vi "PantherLAB_Log - Add New DQMH Module.vi"(4 "New Module Name":string, 6 "New Module Folder":path, 9 "External Module Info":T1, 10 "New Module Type":T3, 11 "Project":refnum<vi>) -> (0 "error out":errorcluster)   [LabVIEW 2016]
doc: "_____\nCreated using DQMH Framework: Event Scripter 7.1.0.1450."
uses:
  <vilib>/Delacor/Delacor QMH/Libraries/_Scripting Support/Module Type (Including External)--enum.ctl
  <vilib>/Delacor/Delacor QMH/Libraries/_Scripting Support/External Module Info--cluster.ctl
  <vilib>/Delacor/Delacor QMH/Libraries/_Scripting Support/Module Type--enum.ctl
  PantherLAB Scripting Hooks/PantherLAB_Log.lvlib
  <vilib>/Delacor/Delacor QMH/Libraries/_Scripting Support/dqmh_lib_DQMH Scripting Support.lvlib
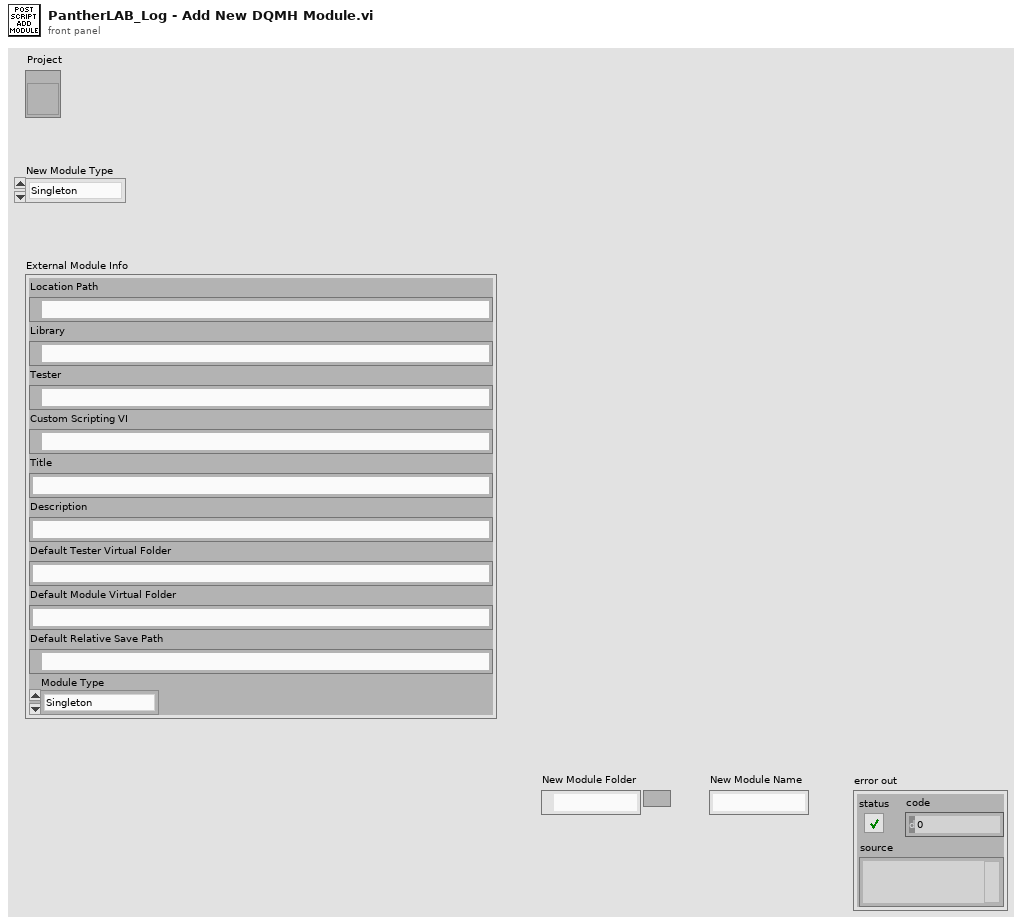
[diagram p1: front panel]
types:
  T1 = typedef "dqmh_lib_DQMH Scripting Support.lvlib/External Module Info--cluster.ctl" = cluster{"Location Path":path, "Library":path, "Tester":path, "Custom Scripting VI":path, "Title":string, "Description":string, "Default Tester Virtual Folder":string, "Default Module Virtual Folder":string, "Default Relative Save Path":path, "Module Type":T2}
  T2 = typedef "dqmh_lib_DQMH Scripting Support.lvlib/Module Type--enum.ctl" = enum16{"Singleton", "Cloneable"}
  T3 = typedef "dqmh_lib_DQMH Scripting Support.lvlib/Module Type (Including External)--enum.ctl" = enum16{"Singleton", "Cloneable", "External"}
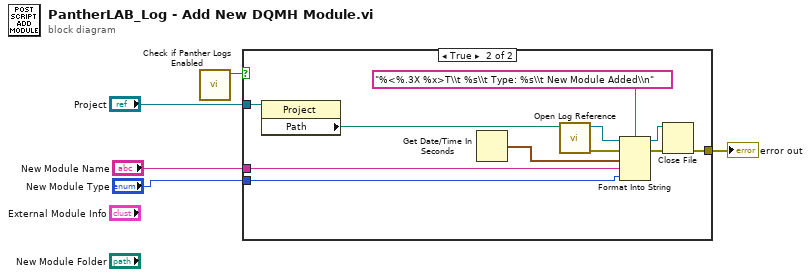
[diagram p0: block diagram]
diagram:
  n1 = call "Check if Panther Logs Enabled.vi"() -> ("PantherLogs Enabled?"=w5:bool)  [unwired: 11 in]
  n2 = case shown="True" w5 {
    tunnel: [_ w14] -> w1
    tunnel: "Project" -> [_ w9]
    tunnel: "New Module Type" -> [_ w7]
    tunnel: "New Module Name" -> [_ w8]
    frame False {
    }
    frame True {
      n3 = property class="Project"(reference=w9) -> ("Path"=w10:path)  [unwired: 1 in, 2 out]
      n4 = Get Date/Time In Seconds() -> (seconds since 1Jan1904=w11:timestamp)
      n5 = call "Open Log Reference.vi"("Project Path"=w10) -> ("error out"=w16:errorcluster, "File Reference"=w13:refnum<file>)  [unwired: 9 in]
      n6 = Format Into String(format string="%<%.3X %x>T\\t %s\\t Type: %s\\t New Module Added\\n", initial string=w13, error in=w16, w11, w8, w7) -> (resulting string=w12:refnum<file>, error out=w15:errorcluster)
      n7 = Close File(refnum=w12, error in=w15) -> (error out=w14:errorcluster)  [unwired: 1 out]
    }
  }
  "error out" <- w1
